vi "DMM_Scan DER Initialize.vi"(0 "Scan Resources Names":T3={"DMM Resource Name"="DMM_4065", "DAQ Resource Physical Channels Names"="PXI_6363/port0/line0:31, PXI_6363/port1/line0:7, PXI_6363/port2/line0:7"}, 2 "Powerline Frequency":T4=enum."50 Hz", 5 "Channels Topology Mapping":T2={"Min Channel Voltage"=0, "Max Channel Voltage"=1, "Min Channel Current"=2, "Max Channel Current"=2, "N Shift Shunt to Min Channel Current"=1} caption="Channels Topology mapping", 7 "Close all Shunts?":bool=TRUE, 9 "Relays Debounce Time (ms)":u32=5, 11 "error in":errorcluster) -> (4 "Scan Resources Handles Out":T1={"DMM Handle"="", "DAQmx Task Out"="", "Relays Status Array"=[FALSE, FALSE, FALSE, TRUE, FALSE, FALSE, FALSE, FALSE, FALSE, FALSE, FALSE, FALSE, FALSE, FALSE, FALSE, FALSE, FALSE, FALSE, FALSE, FALSE, FALSE, FALSE, FALSE, FALSE, FALSE, FALSE, FALSE, FALSE, FALSE, FALSE, FALSE, FALSE, FALSE, FALSE, FALSE, FALSE, FALSE, FALSE, FALSE, FALSE, FALSE, FALSE, FALSE, FALSE, FALSE, FALSE, FALSE, FALSE], "N Shift Shunt"=1, "Close all Shunts?"=TRUE, "Relays Debounce Time (ms)"=5} caption="Scan Resources Handles out", 6 "Topology Mapping Output":string[][](array[string])=[["ch0", "Voltage Type", "PXI_6363/port0/line0"], ["ch1", "Voltage Type", "PXI_6363/port0/line1"], ["ch2", "Current Type ", "PXI_6363/port0/line2"], ["ch3", "Shunt Type linked to ch2", "PXI_6363/port0/line3"], ["ch4", "", "PXI_6363/port0/line4"], ["ch5", "", "PXI_6363/port0/line5"], ["ch6", "", "PXI_6363/port0/line6"], ["ch7", "", "PXI_6363/port0/line7"], ["ch8", "", "PXI_6363/port0/line8"], ["ch9", "", "PXI_6363/port0/line9"], ["ch10", "", "PXI_6363/port0/line10"], ["ch11", "", "PXI_6363/port0/line11"], ["ch12", "", "PXI_6363/port0/line12"], ["ch13", "", "PXI_6363/port0/line13"], ["ch14", "", "PXI_6363/port0/line14"], ["ch15", "", "PXI_6363/port0/line15"], ["ch16", "", "PXI_6363/port0/line16"], ["ch17", "", "PXI_6363/port0/line17"], ["ch18", "", "PXI_6363/port0/line18"], ["ch19", "", "PXI_6363/port0/line19"], ["ch20", "", "PXI_6363/port0/line20"], ["ch21", "", "PXI_6363/port0/line21"], ["ch22", "", "PXI_6363/port0/line22"], ["ch23", "", "PXI_6363/port0/line23"], ["ch24", "", "PXI_6363/port0/line24"], ["ch25", "", "PXI_6363/port0/line25"], ["ch26", "", "PXI_6363/port0/line26"], ["ch27", "", "PXI_6363/port0/line27"], ["ch28", "", "PXI_6363/port0/line28"], ["ch29", "", "PXI_6363/port0/line29"], ["ch30", "", "PXI_6363/port0/line30"], ["ch31", "", "PXI_6363/port0/line31"], ["ch32", "", "PXI_6363/port1/line0"], ["ch33", "", "PXI_6363/port1/line1"], ["ch34", "", "PXI_6363/port1/line2"], ["ch35", "", "PXI_6363/port1/line3"], ["ch36", "", "PXI_6363/port1/line4"], ["ch37", "", "PXI_6363/port1/line5"], ["ch38", "", "PXI_6363/port1/line6"], ["ch39", "", "PXI_6363/port1/line7"], ["ch40", "", "PXI_6363/port2/line0"], ["ch41", "", "PXI_6363/port2/line1"], ["ch42", "", "PXI_6363/port2/line2"], ["ch43", "", "PXI_6363/port2/line3"], ["ch44", "", "PXI_6363/port2/line4"], ["ch45", "", "PXI_6363/port2/line5"], ["ch46", "", "PXI_6363/port2/line6"], ["ch47", "", "PXI_6363/port2/line7"]], 15 "error out":errorcluster)   [LabVIEW 2021, in "DMM_Scan DAQ Ext RLY.lvlib"]
doc: "Creates a new NI-DMM Scan driver session on each device specified in the Scan Resource Names control configured with the local powerline frequency. The device uses the powerline frequency value to select a timebase for setting the Aperture Time property in powerline cycles (PLCs). Change Powerline Frequency value to 60 Hz for North & South America.\n\nYou must declare your custom hardware mapping and topology configuration first. Any DAQ device and port structure can be used including cDAQ relay driver modules and DIO TTL devices (with external amplification). You must declare your positions for the voltage type channels, then the list of current type channels followed by the N-shift position from the first current channel for the shunts. Later, all channels can be scanned randomly on each measurement type, in 2-wire (Differential) configuration. Dual Pole external relays (DPST) are needed for differential measurements attached to each DO line channel. \n\n- \"Close all Shunts\" input is used to close all DAQ DO lines attached to shunt relay channels declared, allowing continuous power delivery to the DUT during all measurements. Deselect \"Close all shunts\" to open current shunts. For example, disable \"Close all shunts\" in the event of a 2-wire resistance measurement function without any current through the DUT.\n\n- Relays Debounce Time (ms), defines the timing specifications for the external relays debounce time. Typical default Value is 5 ms, but needs to be adjusted for your specific choice of external relay. \n\nThe VI returns the Topology Mapping Output to easily check your Mapping declaration and save time to connect the appropriated channel lines of your device. It can help with maintenance and HW modifications.\n\nFor the Shunt channels, the link to the current channel number is returned."
uses:
  DMM_Scan DAQ Ext RLY.lvlib
  <instrlib>/niDMM/nidmm.llb/niDMM Powerline Frequency.ctl
  Typedefs/Scan Resource Names.ctl
  Typedefs/Scan Resource Handles Out.ctl
  DMM Mixed Measurements/DMM_Mixed Measurement.lvlib
  Static Digital State Generation/DAQ_Static Digital State Generation.lvlib
  <resource>/objmgr/daqmx.rc
panel:
  # "Inputs"
  # "Outputs"
  # "Overview:\nThis VI interacts with the NI-DMM and NI-DAQmx drivers to initialize NI-DMM instruments and provide a corresponding instrument handle according to the topology selected. It also provides the fixed hardware mapping topology used by the custom DAQ Multiplexer device ( Ex. PXIe-6363 or NI 6509) you will use.\n\nHardware Requirements: A PXI, PCIe, or USB DMM instrument, and any USB, PCIe, X series or cDAQ device able to control DPST dual independent relays with DO lines pinout.\n\nSoftware Requirements: NI-DMM 2022 Q3 or above, NI-DAQmx 2022 Q4 or above\n\nInstructions:\nSelect your DMM instrument resource name in the drop down control\nSelect your Multiplexer DAQ DO resource from any DAQ board (browse and select the full device name channels/ports)\nSelect and build your Channel Topology Mapping according to your custom external DPST design. Minimum one current and shunt to declare even if they are not used. You can use the VI \"Channels Topology Mapping Tester Tool\" to create and validate your design.\nSelect your Power Line Frequency (Default 50 Hz) and deselect the Close all Shunts? boolean (Default ON) if you don't need to power your DUT through current shunt relays.\n\nNote: each \"DMM Handle Out\" indicator will be used by the Configure & Measure and Close API functions"
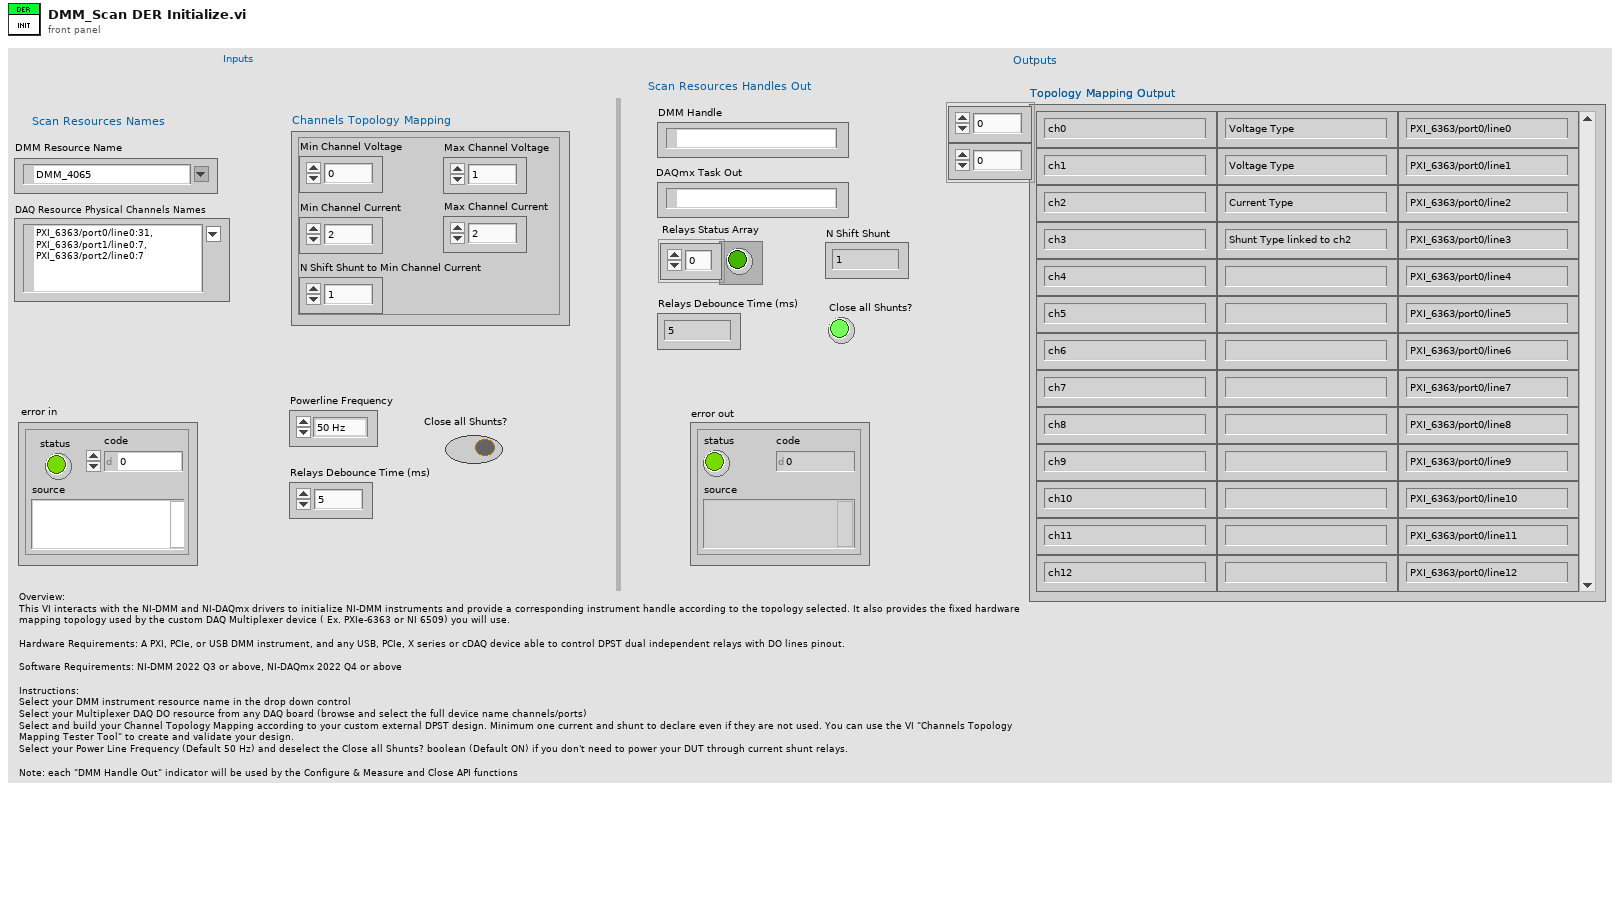
[diagram p1: front panel]
types:
  T1 = typedef "DMM_Scan DAQ Ext RLY.lvlib/Scan Resource Handles Out.ctl" = cluster{"DMM Handle":refnum<k15>, "DAQmx Task Out":refnum<k21>, "Relays Status Array":bool[], "N Shift Shunt":u32, "Close all Shunts?":bool, "Relays Debounce Time (ms)":u32}
  T2 = cluster{"Min Channel Voltage":u32, "Max Channel Voltage":u32, "Min Channel Current":u32, "Max Channel Current":u32, "N Shift Shunt to Min Channel Current":u32}
  T3 = typedef "DMM_Scan DAQ Ext RLY.lvlib/Scan Resource Names.ctl" = cluster{"DMM Resource Name":refnum<k15>, "DAQ Resource Physical Channels Names":tag}
  T4 = typedef "niDMM Powerline Frequency.ctl" = enum16{"60 Hz", "50 Hz"}
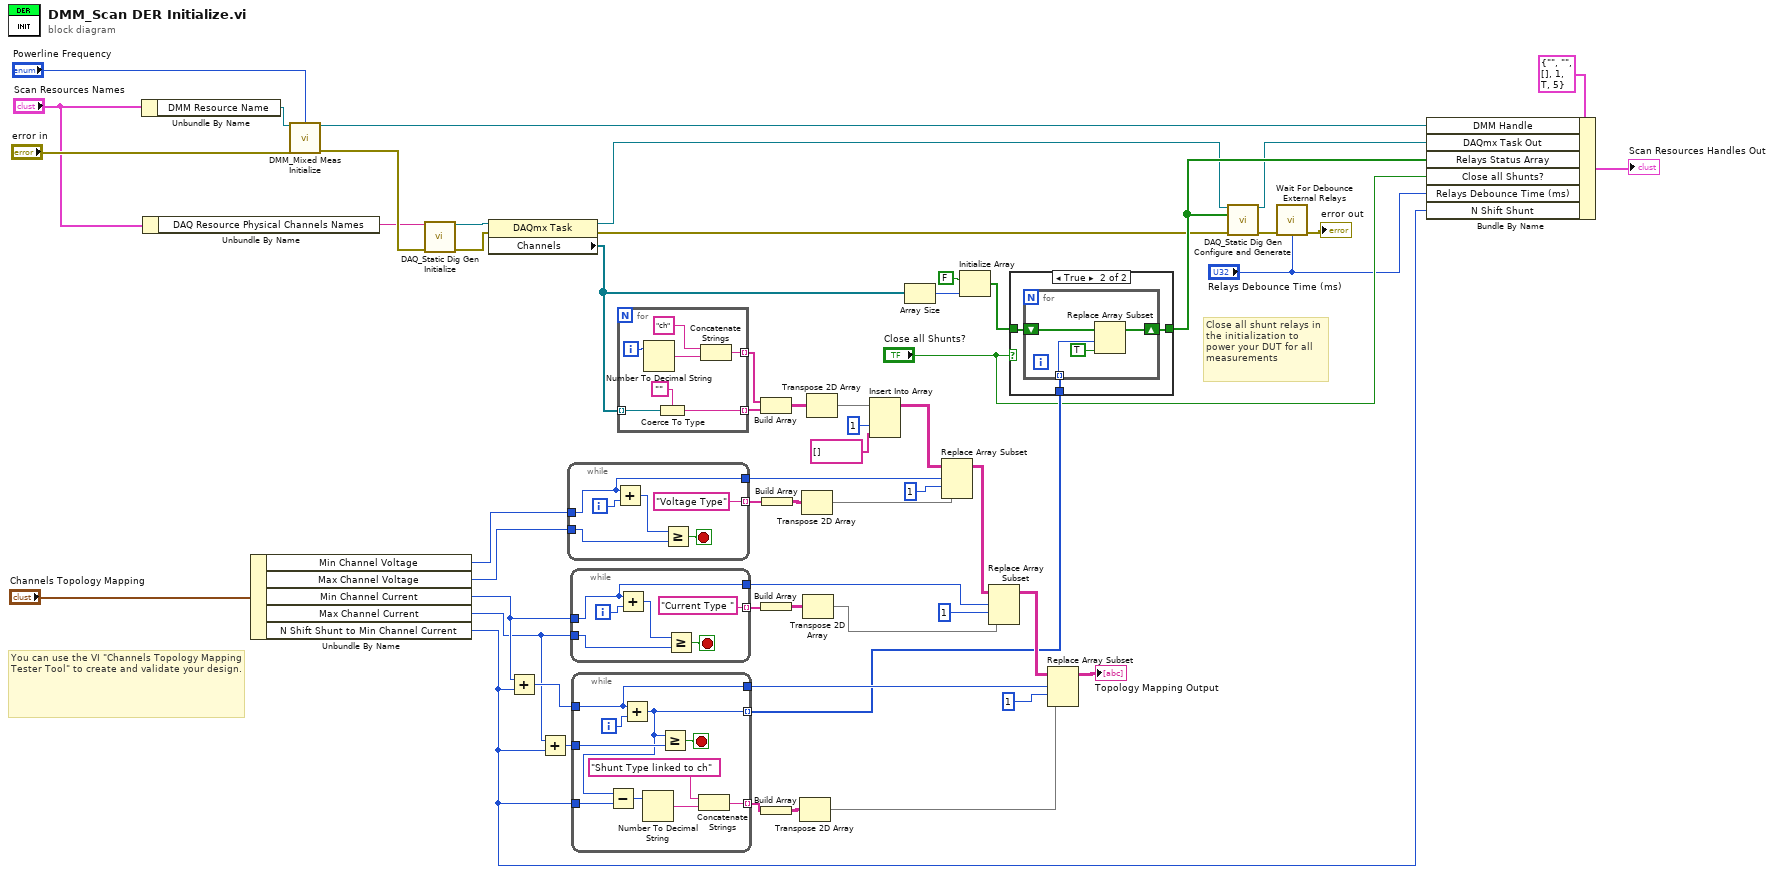
[diagram p0: block diagram]
diagram:
  # "You can use the VI \"Channels Topology Mapping Tester Tool\" to create and validate your design."
  # "Close all shunt relays in the initialization to power your DUT for all measurements"
  n1 = Unbundle By Name("Scan Resources Names") -> ("DMM Resource Name"=w55:refnum<k15>)
  n2 = Unbundle By Name("Scan Resources Names") -> ("DAQ Resource Physical Channels Names"=w51:tag)
  n3 = Unbundle By Name("Channels Topology Mapping") -> ("Min Channel Voltage"=w46:u32, "Max Channel Voltage"=w45:u32, "Min Channel Current"=w33:u32, "Max Channel Current"=w30:u32, "N Shift Shunt to Min Channel Current"=w11:u32)
  n4 = call "DMM_Mixed Meas Initialize.vi"("DMM Resource Name"=w55, "Powerline Frequency"="Powerline Frequency", "error in"="error in") -> ("DMM Handle Out"=w13:refnum<k15>, "error out"=w54:errorcluster)  [unwired: 11 in]
  n5 = call "DAQ_Static Dig Gen Initialize.vi"("Physical Channels"=w51, "error in"=w54) -> ("DAQmx Task Out"=w52:refnum<k21>, "error out"=w50:errorcluster)  [unwired: 12 in]
  n6 = property class="DAQmx Task"(reference=w52, error in=w50) -> (reference out=w4:refnum<k21>, error out=w1:errorcluster, "Channels"=w16:refnum<k21>[])
  n7 = Add(x=w33, y=w11) -> (x+y=w32:u32)
  n8 = Add(x=w30, y=w11) -> (x+y=w31:u32)
  n9 = while {
    tunnel: w46 -> [w58]
    tunnel: w45 -> [w60]
    tunnel: ["Voltage Type"] -> w44 mode=indexing
    tunnel: [w58] -> w40
    i -> [w63]
    stop <- w62 stop-if-true
    n10 = Add(x=w58, y=w63) -> (x+y=w59:u32)
    n11 = Greater Or Equal?(x=w59, y=w60) -> (x >= y?=w62:bool)
  }
  n12 = while {
    tunnel: w33 -> [w64]
    tunnel: w30 -> [w66]
    tunnel: ["Current Type "] -> w38 mode=indexing
    tunnel: [w64] -> w35
    i -> [w69]
    stop <- w68 stop-if-true
    n13 = Add(x=w64, y=w69) -> (x+y=w65:u32)
    n14 = Greater Or Equal?(x=w65, y=w66) -> (x >= y?=w68:bool)
  }
  n15 = while {
    tunnel: w32 -> [w71]
    tunnel: w31 -> [w78]
    tunnel: [w72] -> w24 mode=indexing
    tunnel: [w70] -> w14 mode=indexing
    tunnel: [w71] -> w26
    tunnel: w11 -> [w76]
    i -> [w77]
    stop <- w79 stop-if-true
    n16 = Add(x=w71, y=w77) -> (x+y=w70:u32)
    n17 = Subtract(x=w70, y=w76) -> (x-y=w75:u32)
    n18 = Number To Decimal String(number=w75) -> (decimal integer string=w73:string)  [unwired: 1 in]
    n19 = Greater Or Equal?(x=w70, y=w78) -> (x >= y?=w79:bool)
    n20 = Concatenate Strings("Shunt Type linked to ch", w73) -> (w72:string)
  }
  n21 = for {
    tunnel: w16 -> [w86] mode=indexing
    tunnel: [w85] -> w49 mode=indexing
    tunnel: [w80] -> w48 mode=indexing
    i -> [w83]
    n22 = Number To Decimal String(number=w83) -> (decimal integer string=w82:string)  [unwired: 1 in]
    n23 = Coerce To Type(0:w86, 1:"" ("String Constant")) -> (2:w85:string)
    n24 = Concatenate Strings("ch" ("string"), w82) -> (w80:string)
  }
  n25 = Build Array(w48, w49) -> (w47:string[][])
  n26 = Build Array(w38) -> (w39:string[][])
  n27 = Build Array(w24) -> (w27:string[][])
  n28 = Build Array(w44) -> (w43:string[][])
  n29 = Transpose 2D Array(2D array=w27) -> (transposed array=w29:string[][])
  n30 = Transpose 2D Array(2D array=w43) -> (transposed array=w42:string[][])
  n31 = Transpose 2D Array(2D array=w39) -> (transposed array=w34:string[][])
  n32 = Transpose 2D Array(2D array=w47) -> (transposed array=w22:string[][])
  n33 = Insert Into Array(array=w22, index (col)=1 ("disabled index (col)"), new element=string[] [] ("new element/subarray")) -> (w21:string[][])  [unwired: 1 in]
  n34 = Array Size(array=w16) -> (size(s)=w17:i32)
  n35 = Replace Array Subset(array=w21, new element=w42, index (row)=w40, index (col)=1 ("disabled index (col)")) -> (w36:string[][])
  n36 = Initialize Array(FALSE, w17) -> (w15:bool[])
  n37 = Replace Array Subset(array=w36, new element=w34, index (row)=w35, index (col)=1 ("disabled index (col)")) -> (w25:string[][])
  n38 = case shown="True" "Close all Shunts?" {
    tunnel: w15 -> [w87 w90]
    tunnel: [w87 w89] -> w6
    tunnel: w14 -> [_ w88]
    frame False {
    }
    frame True {
      n39 = for {
        shift-right: [w93] -> w89
        shift-left: w90 -> [w94]
        tunnel: w88 -> [w92] mode=indexing
        n40 = Replace Array Subset(array=w94, new element=TRUE ("new element/subarray"), index=w92) -> (w93:bool[])
      }
    }
  }
  n41 = Replace Array Subset(array=w25, new element=w29, index (row)=w26, index (col)=1 ("disabled index (col)")) -> (→"Topology Mapping Output":string[][])
  n42 = call "DAQ_Static Dig Gen Configure and Generate.vi"("DAQmx Task In"=w4, "Data to Write"=w6, "error in"=w1) -> ("DAQmx Task Out"=w3:refnum<k21>, "error out"=w7:errorcluster)  [unwired: 10 in, 1 out]
  n43 = call "Wait For Debounce External Relays.vi"("error in"=w7, "Wait (ms)"="Relays Debounce Time (ms)") -> ("error out"=→"error out":errorcluster)  [unwired: 13 in]
  n44 = Bundle By Name(cluster=T1 {"DMM Handle"="", "DAQmx Task Out"="", "Relays Status Array"=[], "N Shift Shunt"=1, "Close all Shunts?"=TRUE, "Relays Debounce Time (ms)"=5} ("Scan Resources Handles Out"), "DMM Handle"=w13, "DAQmx Task Out"=w3, "Relays Status Array"=w6, "Close all Shunts?"="Close all Shunts?", "Relays Debounce Time (ms)"="Relays Debounce Time (ms)", "N Shift Shunt"=w11) -> (→"Scan Resources Handles Out":T1)
